vi "Read Log Info.vi"(8 "error in (no error)":errorcluster, 10 "CSV String":string, 11 "VISA resource name":refnum<visa-resource-name>) -> (0 "error out":errorcluster, 2 "Count":i32, 3 "VISA resource name out":refnum<visa-resource-name>)   [LabVIEW 2013, in "Watts Up Series.lvlib"]
doc: "Parses the initial return from the Watts Up device. This contains information about the device. Currently only outputs the count, which is the number of data records on the device."
uses:
  <instrlib>/Watts Up Series/Watts Up Series.lvlib
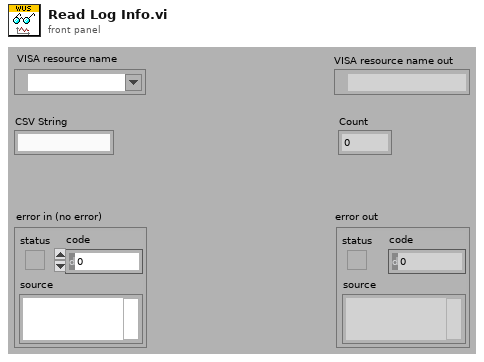
[diagram p1: front panel]
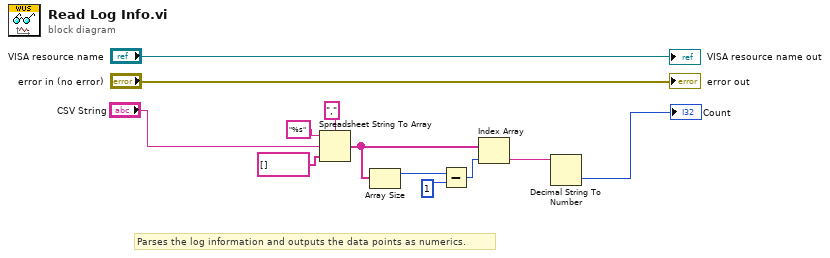
[diagram p0: block diagram]
diagram:
  # "Parses the log information and outputs the data points as numerics."
  n1 = Spreadsheet String To Array(delimiter (Tab)=",", format string="%s", spreadsheet string="CSV String", array type (2D Dbl)=string[] []) -> (array=w1:string[])
  n2 = Array Size(array=w1) -> (size(s)=w8:i32)
  n3 = Subtract(x=w8, y=1) -> (x-y=w10:i32)
  n4 = Index Array(array=w1, index=w10) -> (element=w11:string)
  n5 = Decimal String To Number(string=w11) -> (number=→"Count":i32)  [unwired: 2 in, 1 out]
  "VISA resource name out" <- "VISA resource name"
  "error out" <- "error in (no error)"
